vi "3.1.vi"() -> ()   [LabVIEW 2020]
uses:
  <vilib>/numeric/Random Number (Range) I64.vi
  <vilib>/numeric/sub_Random U32.vi
panel:
  out "°C y filtro":dbl[][](graph)
  out "min index ºC":i32
  out "max value ºC":u64
  out "min index ºF, ºC, FILTRO":i32
  out "max value ºF, ºC, FILTRO":u64
  out "Array":dbl[][](array[numeric])
  out "Valores en °C":i64[](graph)
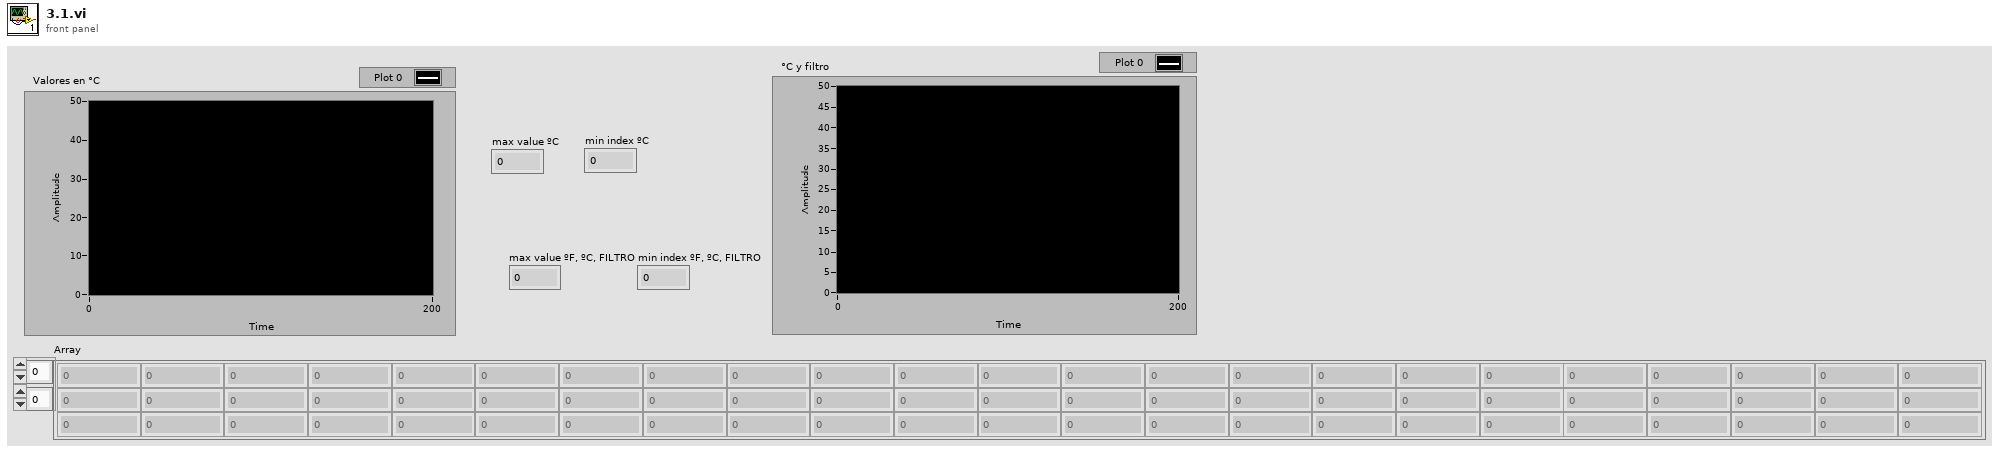
[diagram p1: front panel]
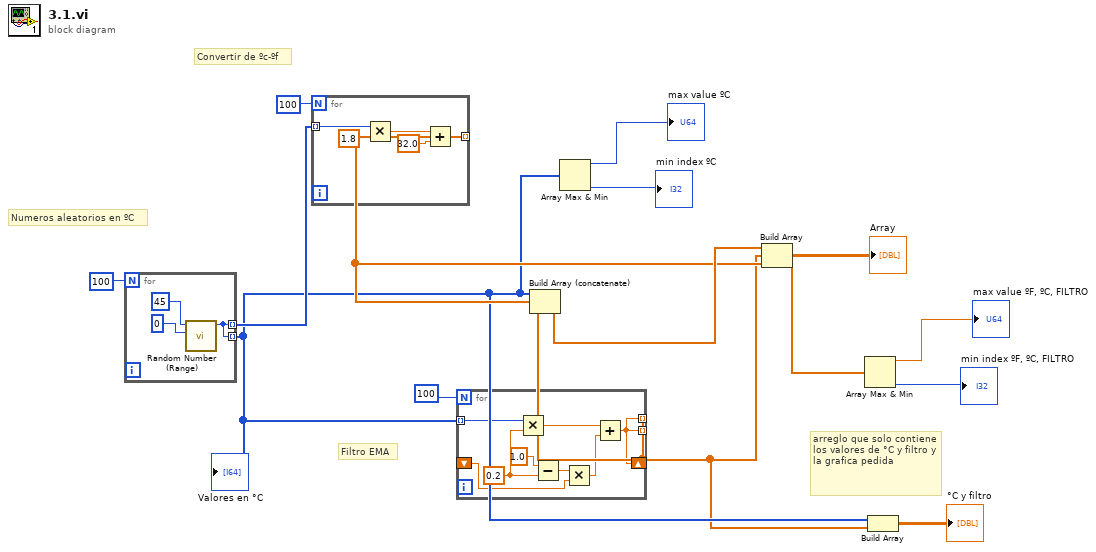
[diagram p0: block diagram]
diagram:
  # "arreglo que solo contiene los valores de °C y filtro y la grafica pedida"
  # "Filtro EMA"
  # "Convertir de ºc-ºf"
  # "Numeros aleatorios en ºC"
  n1 = for {
    N: 100 -> [_]
    tunnel: [w16] -> w3 mode=indexing
    tunnel: [w16] -> w13 mode=indexing
    n2 = call-poly <vilib>:"Random Number (Range).vi"("lower bound (-100)"=u64 0 ("lower bound (0)"), "upper bound (100)"=u64 45) -> ("number"=w16:i64)  [unwired: 9 in]
  }
  "Valores en °C" <- w3
  n3 = for {
    N: 100 -> [_]
    tunnel: w13 -> [w19] mode=indexing
    tunnel: [w18] -> w6 mode=indexing
    n4 = Multiply(x=w19, y=1.8 ("x*y")) -> (x*y=w21:dbl)
    n5 = Add(x=w21, y=32.0) -> (x+y=w18:dbl)
  }
  n6 = for {
    N: 100 -> [_]
    tunnel: w3 -> [w30] mode=indexing
    shift-right: [w23] -> _
    shift-left: _ -> [w24]
    tunnel: [w23] -> _ mode=indexing
    tunnel: [w23] -> w2 mode=indexing
    w28 = 0.2 ("y")
    n7 = Multiply(x=w30, y=w28) -> (x*y=w26:dbl)
    n8 = Subtract(x=1.0, y=w28) -> (x-y=w27:dbl)
    n9 = Multiply(x=w27, y=w24) -> (x*y=w25:dbl)
    n10 = Add(x=w26, y=w25) -> (x+y=w23:dbl)
  }
  n11 = Build Array (concatenate) "Build Array"(w3, w6, w2) -> (w7:dbl[])
  n12 = Array Max & Min(array=w3) -> (max value=→"max value ºC":i64, min index (indices)=→"min index ºC":i32)  [unwired: 2 out]
  n13 = Build Array(w7, w2, w6) -> (→"Array":dbl[][])
  n14 = Array Max & Min(array=w7) -> (max value=→"max value ºF, ºC, FILTRO":dbl, min index (indices)=→"min index ºF, ºC, FILTRO":i32)  [unwired: 2 out]
  n15 = Build Array(w3, w2) -> (→"°C y filtro":dbl[][])
